vi "Highlight row Write.vi"(4 "error in (no error)":errorcluster, 5 "Value":bool, 6 "Container State":T6, 7 "Display State In":T1) -> (0 "error out":errorcluster, 3 "Display State Out":T1)   [LabVIEW 2020, in "KTable.xctl"]
uses:
  KTable.xctl
  <vilib>/_xctls/Container State.ctl
  <vilib>/_xctls/XControlSupport.lvlib
  ColumnType.ctl
  ColumnSpec.ctl
  Table Properties.ctl
  Event Type.ctl
  Event Data.ctl
  Events.ctl
  State.ctl
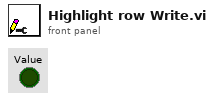
[diagram p1: front panel]
types:
  T1 = typedef "KTable.xctl/State.ctl" = cluster{"Columns":T2[], "Listbox":refnum<vi>, "Default row":string[], "Properties":T4, "Events":T5, "Locked":bool[][], "Size":cluster{"Rows":i32, "Columns":i32}, "rings":i32[][], "DefColors":u32[], "highlight row":bool}
  T2 = typedef "KTable.xctl/ColumnSpec.ctl" = cluster{"Name":string, "Type":T3, "Width":i32, "Strings":string[], "Position":enum16{"Left", "Center", "Right"}, "locked":bool, "cds":cluster{"Strings":string[]}[][], "Hide NaN":bool}
  T3 = typedef "KTable.xctl/ColumnType.ctl" = enum16{"String", "Enum", "Int", "Double", "Boolean", "Ring", "Formula", "Color"}
  T4 = typedef "KTable.xctl/Table Properties.ctl" = cluster{"Vertical scrollbar":bool, "User add/delete":bool, "Max rows":i32, "Row headers":bool}
  T5 = typedef "KTable.xctl/Events.ctl" = cluster{"Items Changed":refnum<user-event>}
  T6 = typedef "XControlSupport.lvlib/Container State.ctl" = cluster{"Indicator?":bool, "Run Mode?":bool, " Refnum":refnum<vi>}
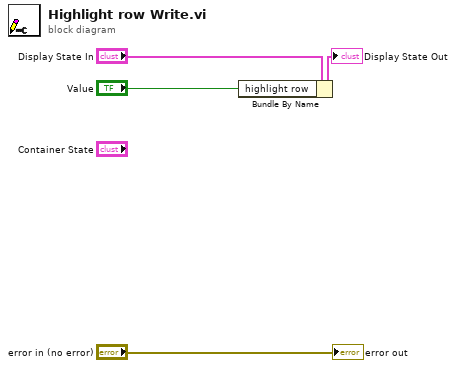
[diagram p0: block diagram]
diagram:
  n1 = Bundle By Name(cluster="Display State In", "highlight row"="Value") -> (→"Display State Out":T1)
  "error out" <- "error in (no error)"
